vi "Calculator.vi"() -> ()   [LabVIEW 2009]
panel:
  in  "Combo Box":string(combo)
  out "Numeric":dbl
  in  "Number 2":dbl
  in  "Number 1":dbl
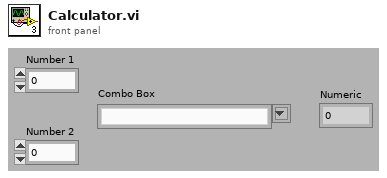
[diagram p1: front panel]
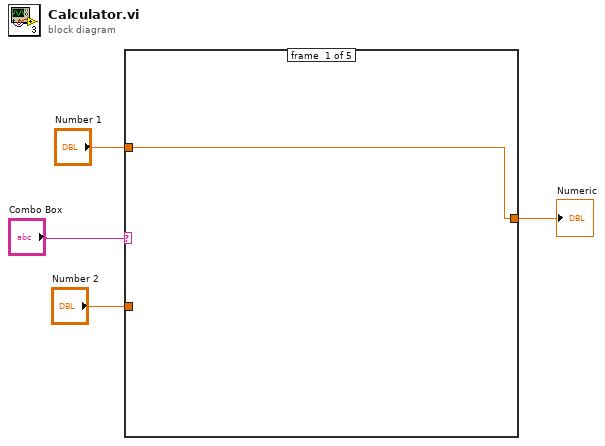
[diagram p0: block diagram]
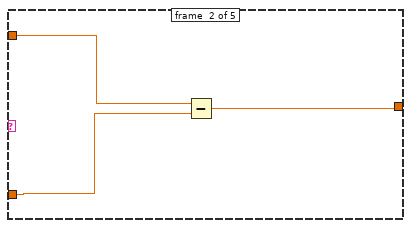
[diagram p2: hidden frame]
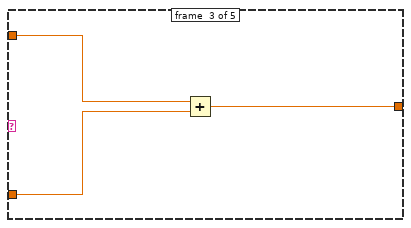
[diagram p3: hidden frame]
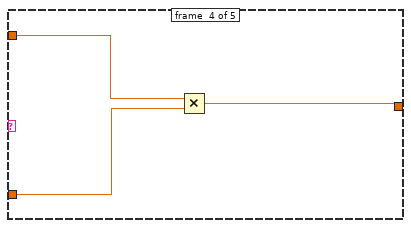
[diagram p4: hidden frame]
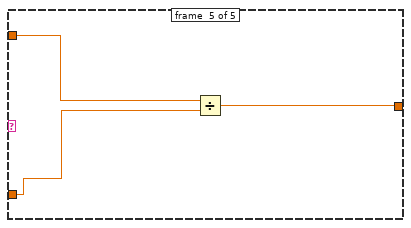
[diagram p5: hidden frame]
diagram:
  n1 = case shown="Default" "Combo Box" {
    tunnel: [w5 w8 w11 w14 w17] -> w4
    tunnel: "Number 1" -> [w5 w7 w9 w13 w16]
    tunnel: "Number 2" -> [_ w6 w10 w12 w15]
    frame #0 {
    }
    frame #1 {
      n2 = Subtract(x=w7, y=w6) -> (x-y=w8:dbl)
    }
    frame #2 {
      n3 = Add(x=w9, y=w10) -> (x+y=w11:dbl)
    }
    frame #3 {
      n4 = Multiply(x=w13, y=w12) -> (x*y=w14:dbl)
    }
    frame #4 {
      n5 = Divide(x=w16, y=w15) -> (x/y=w17:dbl)
    }
  }
  "Numeric" <- w4
